vi "ResizeFacade.vi"   [LabVIEW 2019, in "ExpandVertical.xctl"]
uses:
  ExpandVertical.xctl
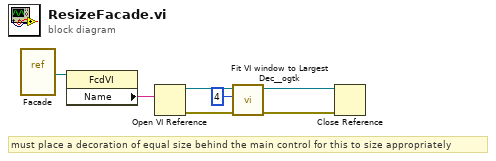
[diagram p0: block diagram]
diagram:
  # "must place a decoration of equal size behind the main control for this to size appropriately"
  n1 = vi-ref "Facade.vi"() -> (w7:refnum<vi>)
  n2 = property class="FcdVI"(reference=w7) -> ("Name"=w6:string)  [unwired: 1 in, 2 out]
  n3 = Open VI Reference(vi path=w6) -> (vi reference=w5:refnum<vi>, error out=w4:errorcluster)  [unwired: 5 in]
  n4 = call <userlib>:"Fit VI window to Largest Dec__ogtk.vi"("error in (no error)"=w4, "border spacing (2 px)"=4, "VI Ref (calling VI)"=w5) -> ("error out"=w2:errorcluster, "dup VI Ref"=w3:refnum<vi>)  [unwired: 3 in]
  n5 = Close Reference(reference=w3, error in (no error)=w2) -> ()  [unwired: 1 out]
